vi "KB-Laser move.vi"(7 "Matches (Geometric Matching 1)":T1[](array[typedef]) {"Correlation Score" format="%.2f"; "Target Template Curve Score" format="%.2f"; "Template Target Curve Score" format="%.2f"; "Bounding Box"."y" format="%.2f"; "Bounding Box"."x" format="%.2f"; "Position"."y" format="%.2f"; "Position"."x" format="%.2f"; "Score" format="%.2f"; "Scale" format="%.2f"; "Angle" format="%.2f"; "Occlusion %" format="%.2f"}, 9 "Fitted Circle (Find Circular Edge 1)":T3 {"Average SNR (dB)" format="%.2f"; "Average Strength" format="%.2f"; "Roundness (Real-World)" format="%.2f"; "Radius (Real-World)" format="%.2f"; "Center (Real-World)"."Y" format="%.2f"; "Center (Real-World)"."X" format="%.2f"; "Radius (Pixels)" format="%.2f"; "Center (Pixels)"."Y" format="%.2f"; "Center (Pixels)"."X" format="%.2f"}, 10 "I roi":T2 {"Contours"."Type" items=["No Selection", "Point", "Line", "Rectangle", "Oval", "Polygon", "Freehand Region", "Annulus", "Unused2", "Unused3", "Broken Line", "Freehand Line", "Rotated Rectangle"]}, 11 "O roi":T2 {"Contours"."Type" items=["No Selection", "Point", "Line", "Rectangle", "Oval", "Polygon", "Freehand Region", "Annulus", "Unused2", "Unused3", "Broken Line", "Freehand Line", "Rotated Rectangle"]}) -> (2 "I roi Out":T2 {"Contours"."Type" items=["No Selection", "Point", "Line", "Rectangle", "Oval", "Polygon", "Freehand Region", "Annulus", "Unused2", "Unused3", "Broken Line", "Freehand Line", "Rotated Rectangle"]}, 3 "O roi Out":T2 {"Contours"."Type" items=["No Selection", "Point", "Line", "Rectangle", "Oval", "Polygon", "Freehand Region", "Annulus", "Unused2", "Unused3", "Broken Line", "Freehand Line", "Rotated Rectangle"]})   [LabVIEW 2015]
uses:
  <vilib>/vision/Pattern Matching.llb/IMAQ GM Match Report.ctl
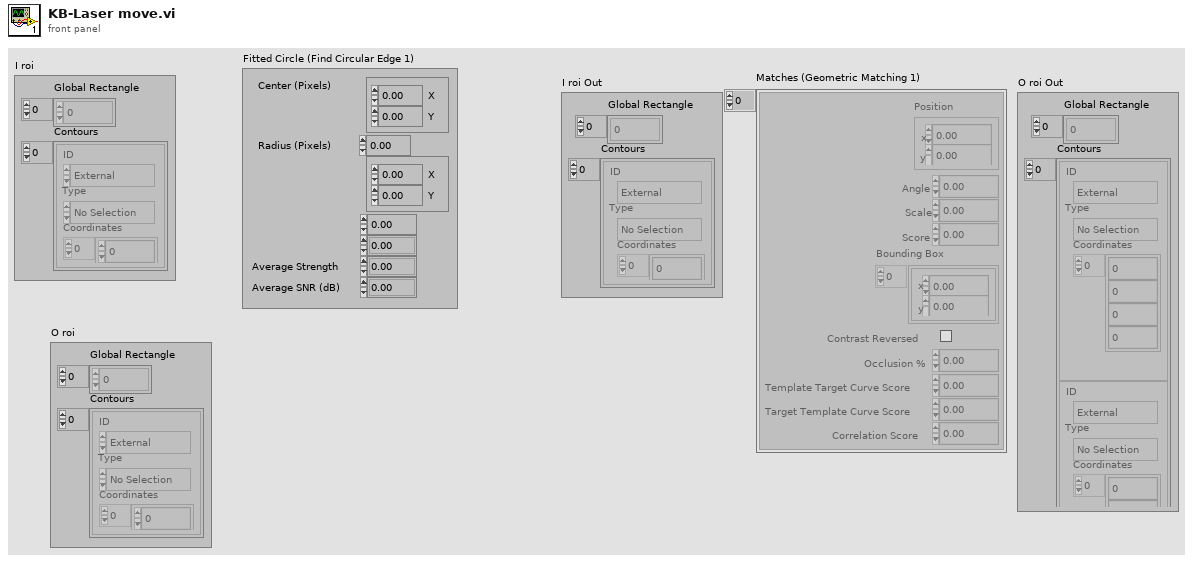
[diagram p1: front panel]
types:
  T1 = typedef "IMAQ GM Match Report.ctl" = cluster{"Position":cluster{"x":sgl, "y":sgl}, "Angle":sgl, "Scale":sgl, "Score":sgl, "Bounding Box":cluster{"x":sgl, "y":sgl}[], "Contrast Reversed":bool, "Occlusion %":sgl, "Template Target Curve Score":sgl, "Target Template Curve Score":sgl, "Correlation Score":sgl}
  T2 = typedef "ROI Descriptor" = cluster{"Global Rectangle":i32[], "Contours":cluster{"ID":enum32{"External", "Internal"}, "Type":u32, "Coordinates":i32[]}[]}
  T3 = cluster{"Center (Pixels)":cluster{"X":sgl, "Y":sgl}, "Radius (Pixels)":dbl, "Center (Real-World)":cluster{"X":sgl, "Y":sgl}, "Radius (Real-World)":dbl, "Roundness (Real-World)":dbl, "Average Strength":dbl, "Average SNR (dB)":dbl}
  T4 = typedef "IMAQ Circle" = cluster{"Center X":i32, "Center Y":i32, "Inner Radius":i32, "Outer Radius":i32, "Start Angle":dbl, "End Angle":dbl}
  T5 = cluster{"ID":enum32{"External", "Internal"}, "Type":u32, "Coordinates":i32[]}[]
  T6 = cluster{"ID":enum32{"External", "Internal"}, "Type":u32, "Coordinates":i32[]}
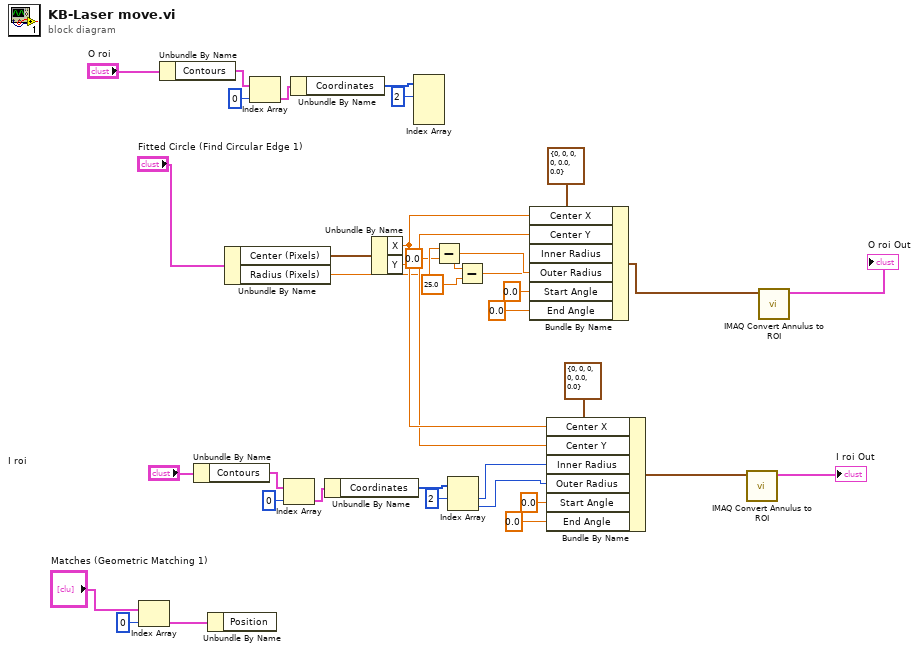
[diagram p0: block diagram]
diagram:
  n1 = Index Array(array="Matches (Geometric Matching 1)", index=0 ("索引")) -> (element=w2:T1)
  n2 = Unbundle By Name("O roi") -> ("Contours"=w32:T5)
  n3 = Unbundle By Name("I roi") -> ("Contours"=w15:T5)
  n4 = Unbundle By Name(w2) -> ()  [unwired: 1 out]
  n5 = Unbundle By Name("Fitted Circle (Find Circular Edge 1)") -> ("Center (Pixels)"=w1:cluster{"X":sgl, "Y":sgl}, "Radius (Pixels)"=w9:dbl)
  n6 = Index Array(array=w32, index=0 ("索引")) -> (element=w30:T6)
  n7 = Index Array(array=w15, index=0 ("索引")) -> (element=w17:T6)
  n8 = Unbundle By Name(w30) -> ("Coordinates"=w29:i32[])
  n9 = Unbundle By Name(w17) -> ("Coordinates"=w18:i32[])
  n10 = Unbundle By Name(w1) -> ("X"=w21:sgl, "Y"=w20:sgl)
  n11 = Index Array(array=w29, index #1=2 ("索引")) -> ()  [unwired: 3 in, 4 out]
  n12 = Subtract(x=w9, y=0.0) -> (x-y=w8:dbl)
  n13 = Index Array(array=w18, index #1=2 ("索引")) -> (element #1=w13:i32, element #2=w12:i32)  [unwired: 1 in]
  n14 = Subtract(x=w8, y=25.0) -> (x-y=w6:dbl)
  n15 = Bundle By Name(cluster=T4 {"Center X"=0, "Center Y"=0, "Inner Radius"=0, "Outer Radius"=0, "Start Angle"=0.0, "End Angle"=0.0} ("Annulus"), "Center X"=w21, "Center Y"=w20, "Inner Radius"=w6, "Outer Radius"=w8, "Start Angle"=0.0, "End Angle"=0.0) -> (w34:T4)
  n16 = Bundle By Name(cluster=T4 {"Center X"=0, "Center Y"=0, "Inner Radius"=0, "Outer Radius"=0, "Start Angle"=0.0, "End Angle"=0.0} ("Annulus"), "Center X"=w21, "Center Y"=w20, "Inner Radius"=w13, "Outer Radius"=w12, "Start Angle"=0.0, "End Angle"=0.0) -> (w11:T4)
  n17 = call "IMAQ Convert Annulus to ROI"("Annulus"=w11) -> ("ROI Descriptor"=→"I roi Out":T2)  [unwired: 8 in, 1 out]
  n18 = call "IMAQ Convert Annulus to ROI"("Annulus"=w34) -> ("ROI Descriptor"=→"O roi Out":T2)  [unwired: 8 in, 1 out]
